vi "send-email.vi"(10 "Message":string, 11 "Recipient Email":string) -> (0 "error out":errorcluster)   [LabVIEW 2019]
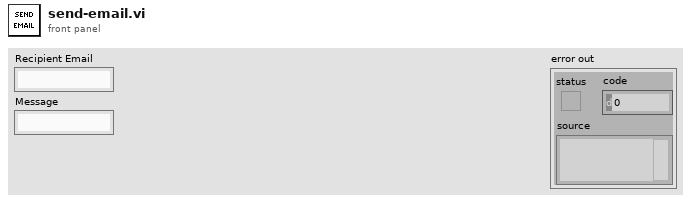
[diagram p1: front panel]
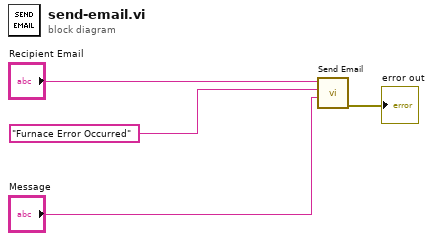
[diagram p0: block diagram]
diagram:
  n1 = call "Send Email"("Message"="Message", "Subject"="Furnace Error Occurred", "Recipients"="Recipient Email") -> ("error out"=→"error out":errorcluster)  [unwired: 8 in]
